vi "Format Help.vi"(8 "error in (no error)":errorcluster, 11 "LV Argument Parser in":refnum<class "LV Argument Parser.lvclass">) -> (0 "error out":errorcluster, 2 "String":string, 3 "LV Argument Parser out":refnum<class "LV Argument Parser.lvclass">)   [LabVIEW 2023, in "LV ArgParse.lvlib" / "LV Argument Parser.lvclass"]
uses:
  LV Argument Parser.lvclass
  LV Argument Parser.lvclass/LV Argument Parser.ctl
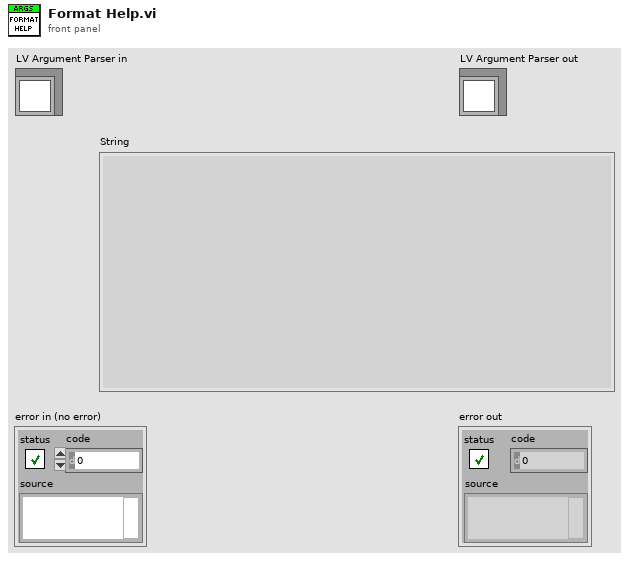
[diagram p1: front panel]
types:
  T1 = typedef "LV ArgParse.lvlib/LV Argument Parser.lvclass/Argument Definition.ctl" = cluster{"Name":string, "short (positional)":string, "long (positional)":string, "action":enum16{"store", "store-const", "store-false", "store-true", "append", "append-const", "count", "help", "version"}, "choices":string[], "const":string, "default":string, "dest (=name)":string, "help":string, "Number":i32, "Required":bool, "Type":enum16{"String", "Int", "Uint", "Float", "Bool", "Date", "Path"}}
  T2 = enum16{"String", "Int", "Uint", "Float", "Bool", "Date", "Path"}
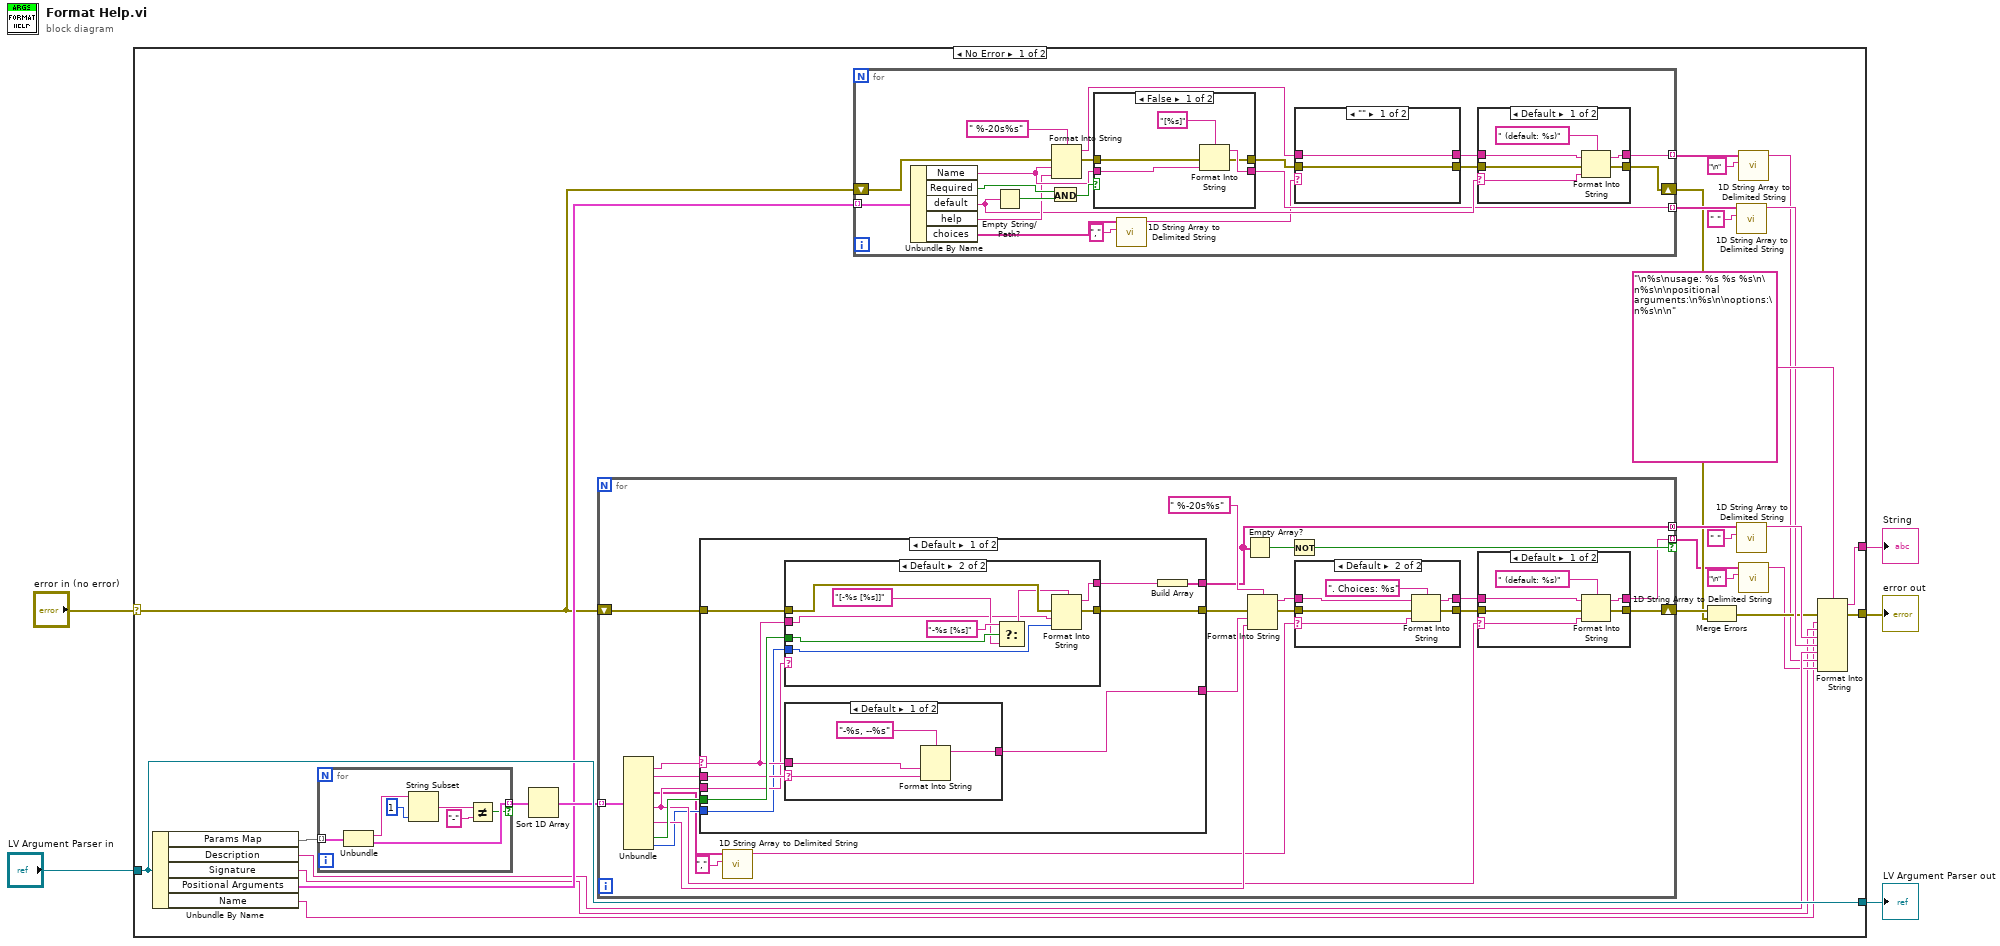
[diagram p0: block diagram]
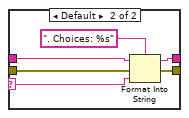
[diagram p2: hidden frame]
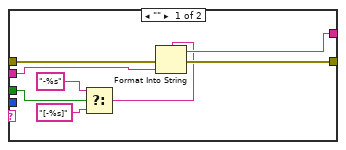
[diagram p7: hidden frame]
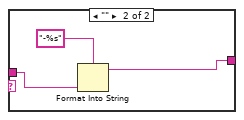
[diagram p8: hidden frame]
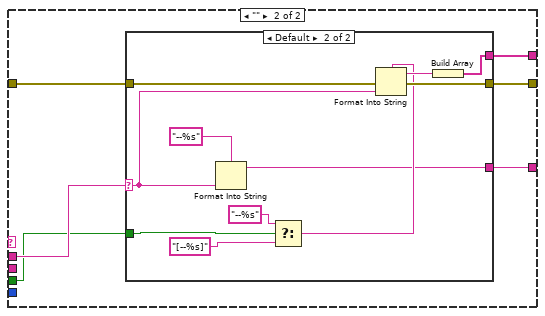
[diagram p9: hidden frame]
diagram:
  n1 = case shown="No Error" "error in (no error)" {
    selector: "error in (no error)" -> [w19 w175]
    tunnel: [w15 w175] -> w4
    tunnel: [w32 w174] -> w2
    tunnel: "LV Argument Parser in" -> [w32 w174]
    tunnel: [w20 _] -> w1
    frame No Error {
      n2 = Unbundle By Name(w32) -> ("Params Map"=w31:map{string, T1}, "Description"=w14:string, "Signature"=w7:string, "Positional Arguments"=w24:T1[], "Name"=w6:string)
      n3 = for {
        tunnel: w31 -> [w173] mode=indexing
        tunnel: [w172] -> w30 mode=indexing if=w167
        n4 = Unbundle(w173) -> (w171:string, "Argument Definition"=w172:T1)
        n5 = String Subset(string=w171, length (rest)=1 ("length (rest)")) -> (substring=w169:string)  [unwired: 1 in]
        n6 = Not Equal?(x=w169, y="-") -> (x != y?=w167:bool)
      }
      n7 = Sort 1D Array(array=w30) -> (sorted array=w29:T1[])
      n8 = for {
        tunnel: w29 -> [w98] mode=indexing
        tunnel: [w90] -> w27 mode=concatenating
        shift-right: [w84] -> w18
        shift-left: w19 -> [w94]
        tunnel: [w86] -> w10 mode=indexing if=w88
        n9 = Unbundle(w98) -> ("short (positional)"=w97:string, "long (positional)"=w96:string, "choices"=w81:string[], "default"=w83:string, "help"=w91:string, "Required"=w95:bool, "Type"=w82:T2)  [unwired: 5 out]
        n10 = case shown="Default" w97 {
          selector: w97 -> [w117 _]
          tunnel: w96 -> [w119 w151]
          tunnel: [w121 w154] -> w90
          tunnel: w94 -> [w123 w153]
          tunnel: [w122 w152] -> w85
          tunnel: w95 -> [w120 w150]
          tunnel: [w118 w149] -> w92
          tunnel: w83 -> [w116 _]
          tunnel: w82 -> [w115 _]
          frame Default {
            n11 = case shown="Default" w116 {
              tunnel: [w131 w140] -> w124
              tunnel: w123 -> [w130 w139]
              tunnel: [w129 w138] -> w122
              tunnel: w120 -> [w127 w136]
              tunnel: w117 -> [w125 w134]
              tunnel: w115 -> [_ w133]
              frame "" {
                n12 = Select(t="-%s" ("format string"), s=w127, f="[-%s]" ("format string")) -> (s? t:f=w128:string)
                n13 = Format Into String(format string=w128, error in=w130, w125) -> (resulting string=w131:string, error out=w129:errorcluster)  [unwired: 1 in]
              }
              frame Default {
                n14 = Select(t="-%s [%s]" ("format string"), s=w136, f="[-%s [%s]]" ("format string")) -> (s? t:f=w137:string)
                n15 = Format Into String(format string=w137, error in=w139, w134, w133) -> (resulting string=w140:string, error out=w138:errorcluster)  [unwired: 1 in]
              }
            }
            n16 = case shown="Default" w119 {
              selector: w119 -> [w143 _]
              tunnel: [w142 w146] -> w118
              tunnel: w117 -> [w144 w147]
              frame Default {
                n17 = Format Into String(format string="-%s, --%s", w144, w143) -> (resulting string=w142:string)  [unwired: 2 in, 1 out]
              }
              frame "" {
                n18 = Format Into String(format string="-%s", w147) -> (resulting string=w146:string)  [unwired: 2 in, 1 out]
              }
            }
            n19 = Build Array(w124) -> (w121:string[])
          }
          frame "" {
            n20 = case shown="Default" w151 {
              selector: w151 -> [_ w157]
              tunnel: [_ w162] -> w154
              tunnel: w153 -> [w155 w164]
              tunnel: [w155 w163] -> w152
              tunnel: w150 -> [_ w160]
              tunnel: [_ w156] -> w149
              frame "" {
              }
              frame Default {
                n21 = Format Into String(format string="--%s", w157) -> (resulting string=w156:string)  [unwired: 2 in, 1 out]
                n22 = Select(t="--%s" ("format string"), s=w160, f="[--%s]" ("format string")) -> (s? t:f=w161:string)
                n23 = Format Into String(format string=w161, error in=w164, w157) -> (resulting string=w165:string, error out=w163:errorcluster)  [unwired: 1 in]
                n24 = Build Array(w165) -> (w162:string[])
              }
            }
          }
        }
        n25 = call <vilib>:"1D String Array to Delimited String.vi"("delimiter"=",", "string array"=w81) -> ("delimited string"=w76:string)  [unwired: 9 in]
        n26 = Empty Array?(array=w90) -> (empty?=w89:bool)
        n27 = Format Into String(format string=" %-20s%s", error in=w85, w92, w91) -> (resulting string=w78:string, error out=w87:errorcluster)  [unwired: 1 in]
        n28 = Not(x=w89) -> (.not. x?=w88:bool)
        n29 = case shown="Default" w76 {
          selector: w76 -> [_ w102]
          tunnel: w87 -> [w99 w106]
          tunnel: [w99 w105] -> w79
          tunnel: w78 -> [w100 w104]
          tunnel: [w100 w103] -> w77
          frame "\u0000" {
          }
          frame Default {
            n30 = Format Into String(format string=". Choices: %s", initial string=w104, error in=w106, w102) -> (resulting string=w103:string, error out=w105:errorcluster)
          }
        }
        n31 = case shown="Default" w83 {
          selector: w83 -> [w109 _]
          tunnel: w77 -> [w112 w113]
          tunnel: [w111 w113] -> w86
          tunnel: w79 -> [w108 w114]
          tunnel: [w107 w114] -> w84
          frame Default {
            n32 = Format Into String(format string=" (default: %s)", initial string=w112, error in=w108, w109) -> (resulting string=w111:string, error out=w107:errorcluster)
          }
          frame "" {
          }
        }
      }
      n33 = for {
        tunnel: w24 -> [w52] mode=indexing
        tunnel: [w40] -> w23 mode=indexing
        shift-right: [w41] -> w16
        shift-left: w19 -> [w48]
        tunnel: [w39] -> w13 mode=indexing
        n34 = Unbundle By Name(w52) -> ("Name"=w45:string, "Required"=w51:bool, "default"=w43:string, "help"=w44:string, "choices"=w37:string[])
        n35 = Empty String/Path?(string/path=w43) -> (empty?=w49:bool)
        n36 = And(x=w51, y=w49) -> (x .and. y?=w50:bool)
        n37 = Format Into String(format string=" %-20s%s", error in=w48, w45, w44) -> (resulting string=w35:string, error out=w47:errorcluster)  [unwired: 1 in]
        n38 = case shown="False" w50 {
          tunnel: [w73 w75] -> w40
          tunnel: w45 -> [w71 w75]
          tunnel: w47 -> [w70 w74]
          tunnel: [w69 w74] -> w42
          frame False {
            n39 = Format Into String(format string="[%s]", error in=w70, w71) -> (resulting string=w73:string, error out=w69:errorcluster)  [unwired: 1 in]
          }
          frame True {
          }
        }
        n40 = call <vilib>:"1D String Array to Delimited String.vi"("delimiter"=",", "string array"=w37) -> ("delimited string"=w33:string)  [unwired: 9 in]
        n41 = case shown="\"\"" w33 {
          selector: w33 -> [_ w55]
          tunnel: w42 -> [w53 w60]
          tunnel: [w53 w59] -> w36
          tunnel: w35 -> [w54 w58]
          tunnel: [w54 w57] -> w34
          frame "" {
          }
          frame Default {
            n42 = Format Into String(format string=". Choices: %s", initial string=w58, error in=w60, w55) -> (resulting string=w57:string, error out=w59:errorcluster)
          }
        }
        n43 = case shown="Default" w43 {
          selector: w43 -> [w63 _]
          tunnel: w34 -> [w66 w67]
          tunnel: [w65 w67] -> w39
          tunnel: w36 -> [w62 w68]
          tunnel: [w61 w68] -> w41
          frame Default {
            n44 = Format Into String(format string=" (default: %s)", initial string=w66, error in=w62, w63) -> (resulting string=w65:string, error out=w61:errorcluster)
          }
          frame "" {
          }
        }
      }
      n45 = Merge Errors(w18, w16) -> (w17:errorcluster)
      n46 = call <vilib>:"1D String Array to Delimited String.vi"("delimiter"=" ", "string array"=w23) -> ("delimited string"=w21:string)  [unwired: 9 in]
      n47 = call <vilib>:"1D String Array to Delimited String.vi"("delimiter"=" ", "string array"=w27) -> ("delimited string"=w25:string)  [unwired: 9 in]
      n48 = call <vilib>:"1D String Array to Delimited String.vi"("delimiter"="\n", "string array"=w13) -> ("delimited string"=w11:string)  [unwired: 9 in]
      n49 = call <vilib>:"1D String Array to Delimited String.vi"("delimiter"="\n", "string array"=w10) -> ("delimited string"=w8:string)  [unwired: 9 in]
      n50 = Format Into String(format string="\n%s\nusage: %s %s %s\n\n%s\n\npositional arguments:\n%s\n\noptions:\n%s\n\n", error in=w17, w6, w7, w25, w21, w14, w11, w8) -> (resulting string=w20:string, error out=w15:errorcluster)  [unwired: 1 in]
    }
    frame Error {
    }
  }
  "error out" <- w4
  "LV Argument Parser out" <- w2
  "String" <- w1
